vi "报警信息.vi"(8 "error in (no error)":errorcluster, 10 "报警信息":string, 11 "设备":string="环境动力") -> (0 "error out":errorcluster)   [LabVIEW 2016, in "采配水.lvlib"]
uses:
  <vilib>/Utility/sysdir.llb/System Directory Type.ctl
  <vilib>/addons/database/Connection.llb/DB Tools Open Connec (String).vi
  <vilib>/addons/database/NI_Database_API.lvlib
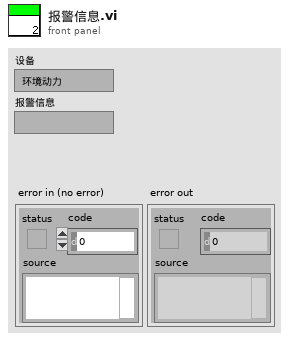
[diagram p1: front panel]
types:
  T1 = typedef "System Directory Type.ctl" = i32
  T2 = cluster{"seconds since 1Jan1904":timestamp, "设备":string, "报警信息":string}
  T3 = typedef "NI_Database_API.lvlib/Conn ObjectReference.ctl" = refnum<k1>
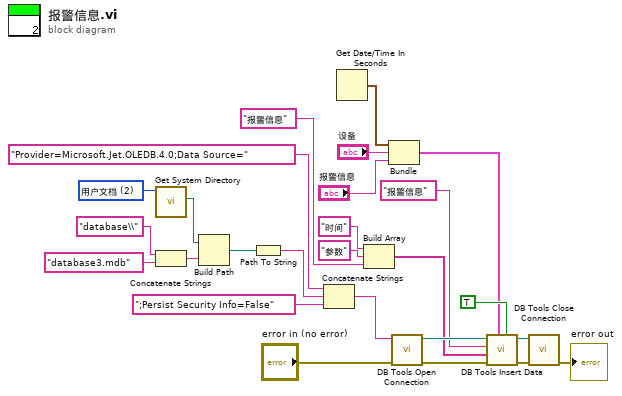
[diagram p0: block diagram]
diagram:
  w20 = T1 2 items=["用户目录"=0, "用户桌面"=1, "用户文档"=2, "用户应用程序数据"=3, "用户设置"=4, "用户临时目录"=5, "公共文档"=6, "公共应用程序数据"=7, "公共设置"=8, "公共缓存"=13, "系统核心库"=9, "系统安装库"=10, "应用程序文件"=11, "启动盘根目录"=12] ("system directory type")
  n1 = call <vilib>:"Get System Directory.vi"("system directory type"=w20) -> ("system directory"=w18:path)  [unwired: 10 in]
  n2 = Concatenate Strings("database\\" ("condition"), "database3.mdb" ("database")) -> (w12:string)
  n3 = Build Path(base path=w18, name or relative path=w12) -> (appended path=w17:path)
  n4 = Path To String(path=w17) -> (string=w16:string)
  n5 = Concatenate Strings("Provider=Microsoft.Jet.OLEDB.4.0;Data Source=" ("condition"), w16, ";Persist Security Info=False" ("condition")) -> (w14:string)
  n6 = Get Date/Time In Seconds() -> (seconds since 1Jan1904=w3:timestamp)
  n7 = Build Array("时间", "参数" ("元素"), "报警信息") -> (w5:string[])
  n8 = Bundle("seconds since 1Jan1904"=w3, "设备"="设备", "报警信息"="报警信息") -> (w4:T2)  [unwired: 1 in]
  n9 = call-poly <vilib>:"DB Tools Open Connection.vi"("error in (no error)"="error in (no error)", "connection information"=w14) -> ("error out"=w10:errorcluster, "connection reference"=w11:T3)  [unwired: 6 in]
  n10 = call <vilib>:"DB Tools Insert Data.vi"("create table? (F)"=TRUE, "data"=w4, "error in (no error)"=w10, "columns"=w5, "table"="报警信息", "connection reference"=w11) -> ("error out"=w22:errorcluster, "connection reference out"=w23:T3)  [unwired: 4 in]
  n11 = call <vilib>:"DB Tools Close Connection.vi"("error in (no error)"=w22, "connection reference"=w23) -> ("error out"=→"error out":errorcluster)  [unwired: 5 in]
